vi "ZP.vi"(8 "error in (no error)":errorcluster, 10 "Axis Number":i32, 11 "Agilis in":T1) -> (0 "error out":errorcluster, 3 "Agilis out":T1)   [LabVIEW 2016, in "Drivers.lvlib" / "Agilis.lvlib"]
doc: "This command is specific to AG-UC8. The piezo actuators are selected by paris which are grouped in four channels. This command <b>changes</b> the selected channel."
uses:
  Agilis.lvlib
  AgilisCmdLib Refnum.ctl
  D:/Trace Grabber/Drivers/Agilis/AgilisCmdLib.dll
  AgilisCmdLib.dll
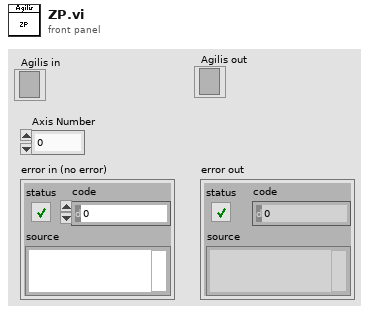
[diagram p1: front panel]
types:
  T1 = typedef "Drivers.lvlib/Agilis.lvlib/AgilisCmdLib Refnum.ctl" = refnum<k24>
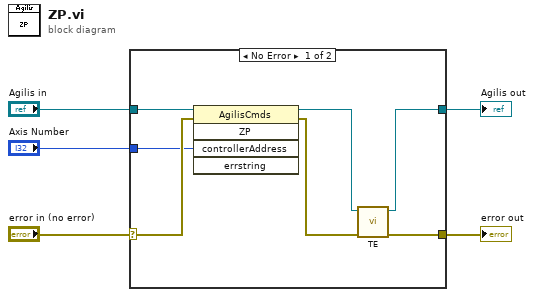
[diagram p0: block diagram]
diagram:
  n1 = case shown="No Error" "error in (no error)" {
    selector: "error in (no error)" -> [w11 w14]
    tunnel: "Agilis in" -> [w12 w13]
    tunnel: [w6 w13] -> w3
    tunnel: [w8 w14] -> w2
    tunnel: "Axis Number" -> [w10 _]
    frame No Error {
      n2 = invoke class="AgilisCmds" method="ZP"(reference=w12, error in=w11, "controllerAddress"=w10) -> (reference out=w7:T1, error out=w9:errorcluster)  [unwired: 2 in, 3 out]
      n3 = call "TE.vi"("error in (no error)"=w9, "Agilis in"=w7) -> ("error out"=w8:errorcluster, "Agilis out"=w6:T1)  [unwired: 8 in]
    }
    frame Error {
    }
  }
  "Agilis out" <- w3
  "error out" <- w2
